vi "Cluster - Read Age.vi"(8 "error in (no error)":errorcluster, 11 "ClusterWithClass":T1) -> (0 "error out":errorcluster, 3 "ClusterWithClass Out":T1)   [LabVIEW 2012]
uses:
  ClassDefinitions/SimpleClassWithProperties/myClass.lvclass
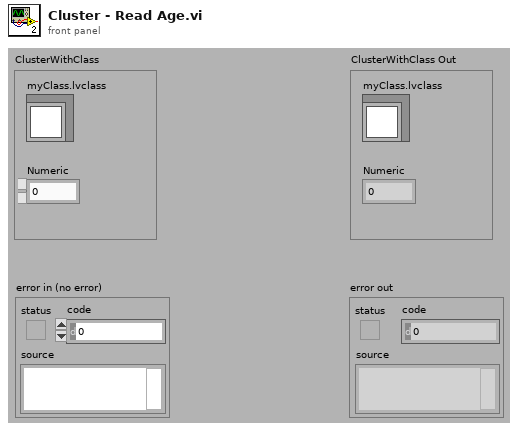
[diagram p1: front panel]
types:
  T1 = cluster{"myClass.lvclass":refnum<class "myClass.lvclass">, "Numeric":dbl}
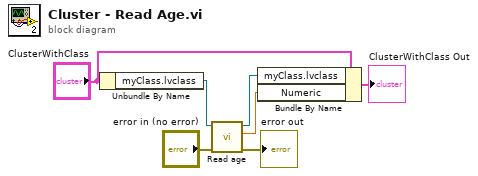
[diagram p0: block diagram]
diagram:
  n1 = Unbundle By Name("ClusterWithClass") -> ("myClass.lvclass"=w7:refnum<class "myClass.lvclass">)
  n2 = call-dynamic "Read age.vi"("error in (no error)"="error in (no error)", "myClass in"=w7) -> ("error out"=→"error out":errorcluster, "age"=w1:dbl, "myClass out"=w4:refnum<class "myClass.lvclass">)  [unwired: 7 in]
  n3 = Bundle By Name(cluster="ClusterWithClass", "myClass.lvclass"=w4, "Numeric"=w1) -> (→"ClusterWithClass Out":T1)
